vi "LIDAR Line mux.vi"(8 "Lines In":T1(array[cluster]) {"End Point"."Y" format="%.2f"; "End Point"."X" format="%.2f"; "Start Point"."Y" format="%.2f"; "Start Point"."X" format="%.2f"}, 10 "Angle In":dbl[](array[numeric]), 11 "Range In":dbl[](array[numeric])) -> (2 "Angle Out":dbl[](array[numeric]), 3 "Range Out":dbl[](array[numeric]))   [LabVIEW 2011]
uses:
  Robot Parameters/Robot Parameters.vi
  <vilib>/Analysis/coordinate.llb/2D Cartesian Coordinate Rotation (Scalar).vi
  <vilib>/Analysis/NI_AALPro.lvlib
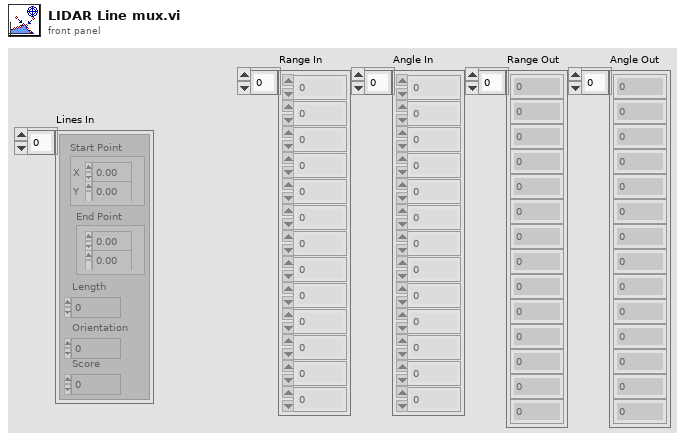
[diagram p1: front panel]
types:
  T1 = cluster{"Start Point":cluster{"X":sgl, "Y":sgl}, "End Point":cluster{"X":sgl, "Y":sgl}, "Length":dbl, "Orientation":dbl, "Score":dbl}[]
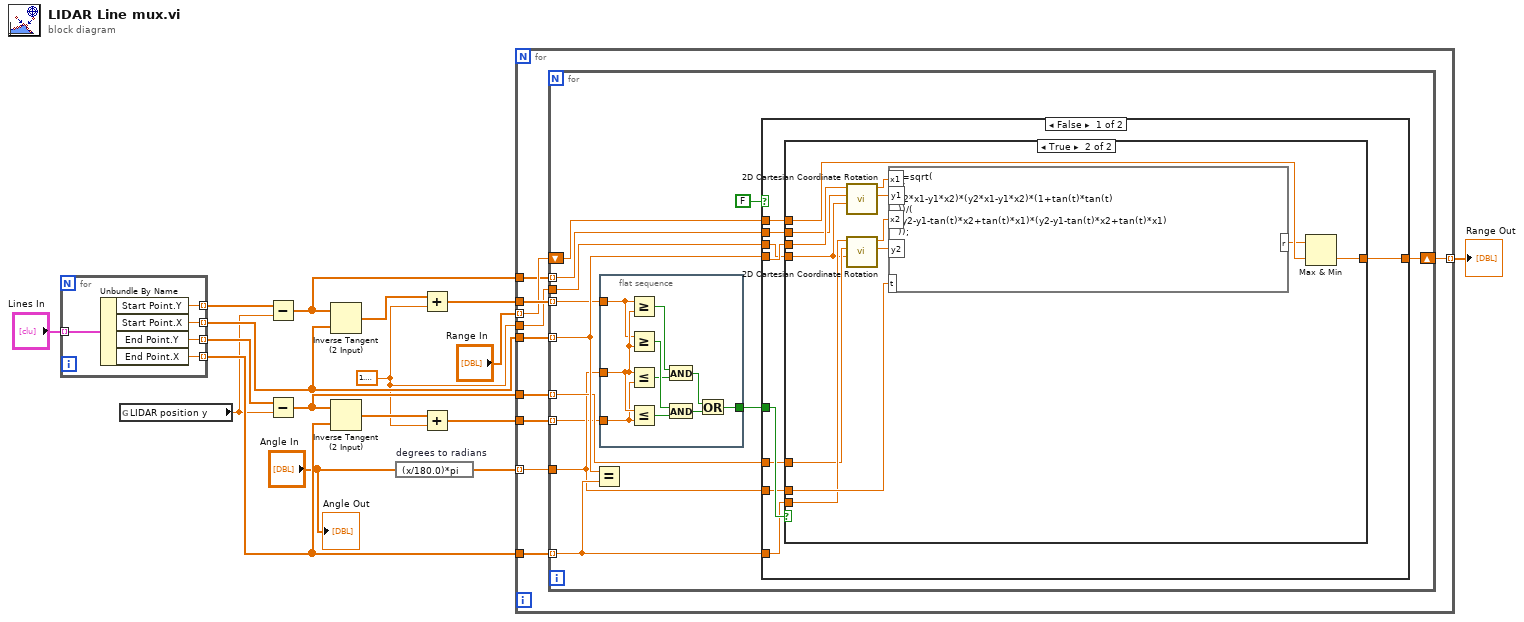
[diagram p0: block diagram]
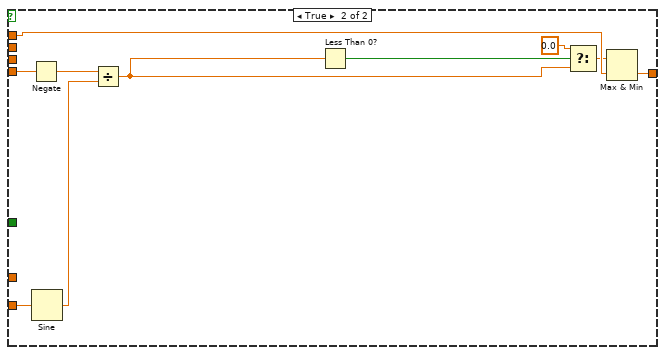
[diagram p3: hidden frame]
diagram:
  w2 = 1.5707963267948966
  n1 = for {
    tunnel: "Lines In" -> [w22] mode=indexing
    tunnel: [w21] -> w11 mode=indexing
    tunnel: [w20] -> w13 mode=indexing
    tunnel: [w19] -> w9 mode=indexing
    tunnel: [w18] -> w12 mode=indexing
    n2 = Unbundle By Name(w22) -> ("Start Point.Y"=w21:sgl, "Start Point.X"=w20:sgl, "End Point.Y"=w19:sgl, "End Point.X"=w18:sgl)
  }
  n3 = global read "Robot Parameters.vi" "LIDAR position y"() -> (w3:dbl)
  n4 = Subtract(x=w11, y=w3) -> (x-y=w10:dbl[])
  n5 = Subtract(x=w9, y=w3) -> (x-y=w8:dbl[])
  n6 = Inverse Tangent (2 Input)(1:w13, 2:w10) -> (0:w7:dbl[])
  n7 = Inverse Tangent (2 Input)(1:w12, 2:w8) -> (0:w5:dbl[])
  n8 = expression code="(x/180.0)*pi" "degrees to radians"("Angle In") -> (w16:dbl[])
  n9 = Add(x=w7, y=w2) -> (x+y=w6:dbl[])
  n10 = Add(x=w5, y=w2) -> (x+y=w4:dbl[])
  n11 = for {
    tunnel: w6 -> [w32]
    tunnel: w4 -> [w31]
    tunnel: w16 -> [w28] mode=indexing
    tunnel: [w30] -> w15 mode=indexing
    tunnel: "Range In" -> [w29] mode=indexing
    tunnel: w13 -> [w27]
    tunnel: w10 -> [w26]
    tunnel: w8 -> [w25]
    tunnel: w12 -> [w24]
    tunnel: w2 -> [w23]
    n12 = for {
      tunnel: w32 -> [w37] mode=indexing
      tunnel: w31 -> [w36] mode=indexing
      shift-right: [w44] -> w30
      shift-left: w29 -> [w43]
      tunnel: w28 -> [w38]
      tunnel: w27 -> [w42] mode=indexing
      tunnel: w26 -> [w41] mode=indexing
      tunnel: w25 -> [w40] mode=indexing
      tunnel: w24 -> [w39] mode=indexing
      tunnel: w23 -> [w33]
      n13 = Equal?(x=w42, y=w39) -> ()  [unwired: 1 out]
      n14 = flat-sequence {
        tunnel: w38 -> [w48]
        tunnel: w37 -> [w47]
        tunnel: w36 -> [w46]
        tunnel: [w45] -> w34
        frame #0 {
          n15 = Greater Or Equal?(x=w47, y=w48) -> (x >= y?=w50:bool)
          n16 = Greater Or Equal?(x=w47, y=w48) -> (x >= y?=w54:bool)
          n17 = Less Or Equal?(x=w48, y=w46) -> (x <= y?=w49:bool)
          n18 = Less Or Equal?(x=w48, y=w46) -> (x <= y?=w53:bool)
          n19 = And(x=w50, y=w49) -> (x .and. y?=w51:bool)
          n20 = And(x=w54, y=w53) -> (x .and. y?=w52:bool)
          n21 = Or(x=w51, y=w52) -> (x .or. y?=w45:bool)
        }
      }
      n22 = case shown="False" FALSE {
        tunnel: w34 -> [w63 _]
        tunnel: [w62 w83] -> w44
        tunnel: w43 -> [w61 w84]
        tunnel: w42 -> [w56 w87]
        tunnel: w41 -> [w60 _]
        tunnel: w40 -> [w59 _]
        tunnel: w39 -> [w58 _]
        tunnel: w38 -> [w57 w82]
        tunnel: w33 -> [w55 _]
        frame False {
          n23 = case shown="True" w63 {
            tunnel: [w64 w77] -> w62
            tunnel: w61 -> [w64 w76]
            tunnel: w60 -> [_ w72]
            tunnel: w59 -> [_ w66]
            tunnel: w58 -> [_ w69]
            tunnel: w57 -> [_ w75]
            tunnel: w56 -> [_ w73]
            tunnel: w55 -> [_ w65]
            frame False {
            }
            frame True {
              n24 = call-poly <vilib>:"2D Cartesian Coordinate Rotation.vi"("theta"=w65, "y"=w72, "x"=w73) -> ("y out"=w70:dbl, "x out"=w71:dbl)  [unwired: 6 in, 1 out]
              n25 = call-poly <vilib>:"2D Cartesian Coordinate Rotation.vi"("theta"=w65, "y"=w66, "x"=w69) -> ("y out"=w67:dbl, "x out"=w68:dbl)  [unwired: 6 in, 1 out]
              n26 = formula code="r=sqrt(\n((\ny2*x1-y1*x2)*(y2*x1-y1*x2)*(1+tan(t)*tan(t)\n))/(\n(y2-y1-tan(t)*x2+tan(t)*x1)*(y2-y1-tan(t)*x2+tan(t)*x1)\n));"("x2"=w68, "y2"=w67, "t"=w75, "x1"=w71, "y1"=w70) -> ("r"=w74:dbl)
              n27 = Max & Min(x=w74, y=w76) -> (min(x,y)=w77:dbl)  [unwired: 1 out]
            }
          }
        }
        frame True {
          n28 = Negate(x=w87) -> (-x=w86:sgl)
          n29 = Sine(x=w82) -> (sin(x)=w85:dbl)
          n30 = Divide(x=w86, y=w85) -> (x/y=w79:dbl)
          n31 = Less Than 0?(x=w79) -> (x < 0?=w81:bool)
          n32 = Select(t=0.0, s=w81, f=w79) -> (s? t:f=w78:dbl)
          n33 = Max & Min(x=w78, y=w84) -> (min(x,y)=w83:dbl)  [unwired: 1 out]
        }
      }
    }
  }
  "Range Out" <- w15
  "Angle Out" <- "Angle In"
